vi "_Prune.vi"(8 "Error In":errorcluster, 10 "Maximum File Index":i32, 11 "File In":refnum<file>) -> (0 "Error Out":errorcluster, 3 "File Out":refnum<file>)   [LabVIEW 2015, in "Logger.lvlib" / "File.lvlib"]
uses:
  File.lvlib
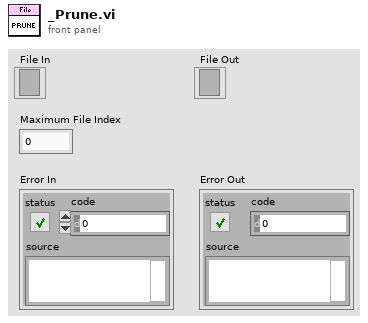
[diagram p1: front panel]
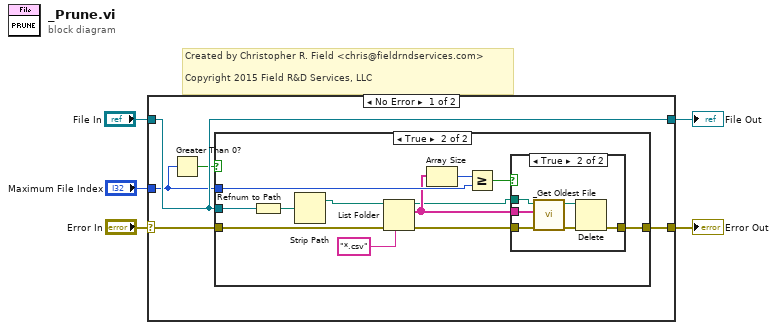
[diagram p0: block diagram]
diagram:
  # "Created by Christopher R. Field <chris@fieldrndservices.com>\n\nCopyright 2015 Field R&D Services, LLC"
  n1 = case shown="No Error" "Error In" {
    selector: "Error In" -> [w10 w32]
    tunnel: "File In" -> [w8 w31]
    tunnel: "Maximum File Index" -> [w7 _]
    tunnel: [w9 w32] -> w2
    tunnel: [w8 w31] -> w1
    frame No Error {
      n2 = Greater Than 0?(x=w7) -> (x > 0?=w6:bool)
      n3 = case shown="True" w6 {
        tunnel: w10 -> [w11 w20]
        tunnel: w7 -> [_ w18]
        tunnel: [w11 w13] -> w9
        tunnel: w8 -> [_ w12]
        frame False {
        }
        frame True {
          n4 = Refnum to Path(1:w12) -> (0:w23:path)
          n5 = Strip Path(path=w23) -> (stripped path=w22:path)  [unwired: 1 out]
          n6 = List Folder(path=w22, pattern="*.csv", error in=w20) -> (path out=w14:path, filenames=w15:string[], error out=w16:errorcluster)  [unwired: 1 in, 1 out]
          n7 = Array Size(array=w15) -> (size(s)=w19:i32)
          n8 = Greater Or Equal?(x=w19, y=w18) -> (x >= y?=w17:bool)
          n9 = case shown="True" w17 {
            tunnel: w16 -> [w24 w30]
            tunnel: w15 -> [_ w28]
            tunnel: w14 -> [_ w29]
            tunnel: [w24 w25] -> w13
            frame False {
            }
            frame True {
              n10 = call "_Get Oldest File.vi"("Error In"=w30, "File Names"=w28, "Folder"=w29) -> ("Error Out"=w26:errorcluster, "Oldest File"=w27:path)  [unwired: 7 in]
              n11 = Delete(path (use dialog)=w27, error in=w26) -> (error out=w25:errorcluster)  [unwired: 3 in, 2 out]
            }
          }
        }
      }
    }
    frame Error {
    }
  }
  "Error Out" <- w2
  "File Out" <- w1
